vi "isEmpty.vi"(8 "error in (no error)":errorcluster, 11 "Bucket in":refnum<class "Bucket.lvclass">) -> (0 "error out":errorcluster, 2 "Empty?":bool, 3 "Bucket out":refnum<class "Bucket.lvclass">)   [LabVIEW 2017, in "Bucket.lvclass"]
uses:
  <userlib>/836-Library/Data_Structures/HashMap/Support/Bucket/Bucket.lvclass
  <userlib>/836-Library/Data_Structures/HashMap/Support/Bucket/Bucket.lvclass/Bucket.ctl
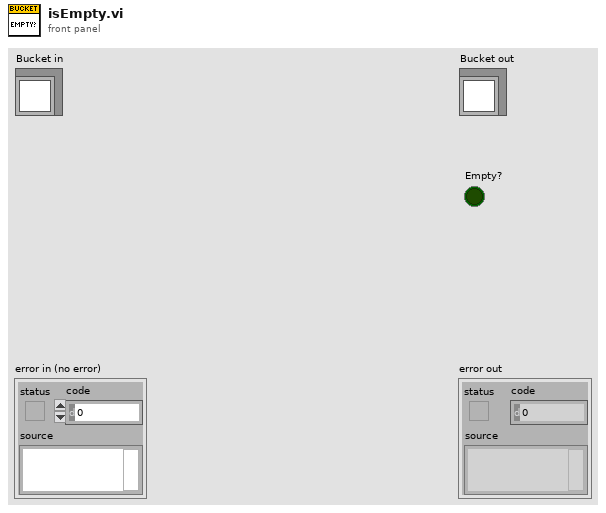
[diagram p1: front panel]
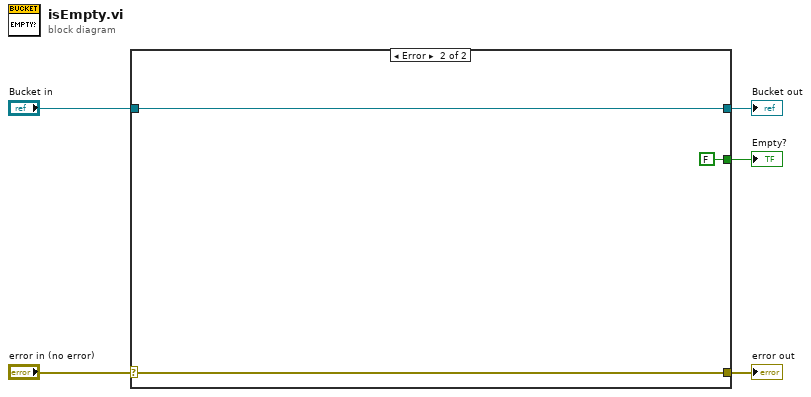
[diagram p0: block diagram]
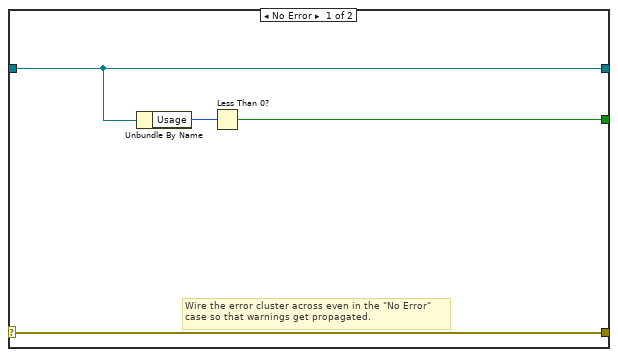
[diagram p2: hidden frame]
diagram:
  n1 = case shown="Error" "error in (no error)" {
    selector: "error in (no error)" -> [w9 w12]
    tunnel: [w9 w12] -> w4
    tunnel: [w8 w11] -> w2
    tunnel: "Bucket in" -> [w8 w11]
    tunnel: [w6 FALSE] -> w1
    frame No Error {
      # "Wire the error cluster across even in the \"No Error\"\ncase so that warnings get propagated."
      n2 = Unbundle By Name(w8) -> ("Usage"=w7:u32)
      n3 = Less Than 0?(x=w7) -> (x < 0?=w6:bool)
    }
    frame Error {
    }
  }
  "error out" <- w4
  "Bucket out" <- w2
  "Empty?" <- w1
